vi "Voltage.vi"(1 "volt":dbl format="%.2f") -> (0 "Command_ str":string)   [LabVIEW 2022 SP3]
panel:
  out "steps":dbl format="%.2f"
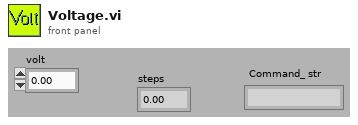
[diagram p1: front panel]
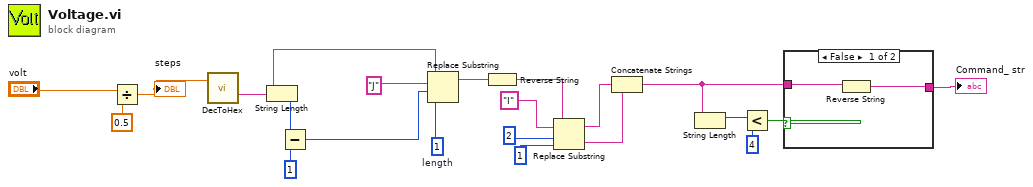
[diagram p0: block diagram]
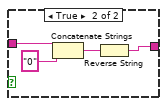
[diagram p2: hidden frame]
diagram:
  w18 = 1  # length
  n1 = Divide(x="volt", y=0.5) -> (x/y=w20:dbl)
  "steps" <- w20
  n2 = call "DecToHex.vi"("Decimal . Decimal Representation"=w20) -> ("HEX . HEX representation"=w19:string)  [unwired: 1 out]
  n3 = String Length(string=w19) -> (length=w16:i32)
  n4 = Subtract(x=w16, y=1) -> (x-y=w3:i32)
  n5 = Replace Substring(2:w18, 3:w3, 4:"J", 5:w19) -> (1:w15:string)  [unwired: 1 out]
  n6 = Reverse String(1:w15) -> (0:w14:string)
  n7 = Replace Substring(2:1, 3:2, 4:"I", 5:w14) -> (0:w9:string, 1:w10:string)
  n8 = Concatenate Strings(w10, w9) -> (w6:string)
  n9 = String Length(string=w6) -> (length=w8:i32)
  n10 = Less?(x=w8, y=4) -> (x < y?=w5:bool)
  n11 = case shown="False" w5 {
    tunnel: w6 -> [w23 w26]
    tunnel: [w22 w24] -> w4
    frame False {
      n12 = Reverse String(1:w23) -> (0:w22:string)
    }
    frame True {
      n13 = Concatenate Strings(w26, "0") -> (w25:string)
      n14 = Reverse String(1:w25) -> (0:w24:string)
    }
  }
  "Command_ str" <- w4
